vi "FTW-Test-Socket-Stress-InboxConnector.vi"() -> (0 "Test Result":errorcluster)   [LabVIEW 2014]
uses:
  src/core/socket/support/FTW-Socket-Core-TransportScheme.ctl
  src/core/error/FTW-ERR-ExceptionType.ctl
  src/core/error/FTW-ERR-Assert-DeveloperError.vi
  src/core/error/FTW-ERR-ThrowError.vi
  src/core/error/FTW-ERR-CallChain.vi
  src/core/string/FTW-STR-ReplaceWhitespace.vi
panel:
  in  "Mode":enum32{"Automated Testing", "Manual Control"}(tab)
  out "Progress":dbl(slide) scale=0.0..1.0
  in  "Test to Perform":T1(radio)=enum."Parallel: 10x100x10k"
  in  "stop":bool
  out "Results":T3(array[cluster]) {"?" format="%_3p bytes/sec (one-way receive)"; "?" format="%_3f replies/sec"; "?" format="Benchmark Time: %_3psec"}
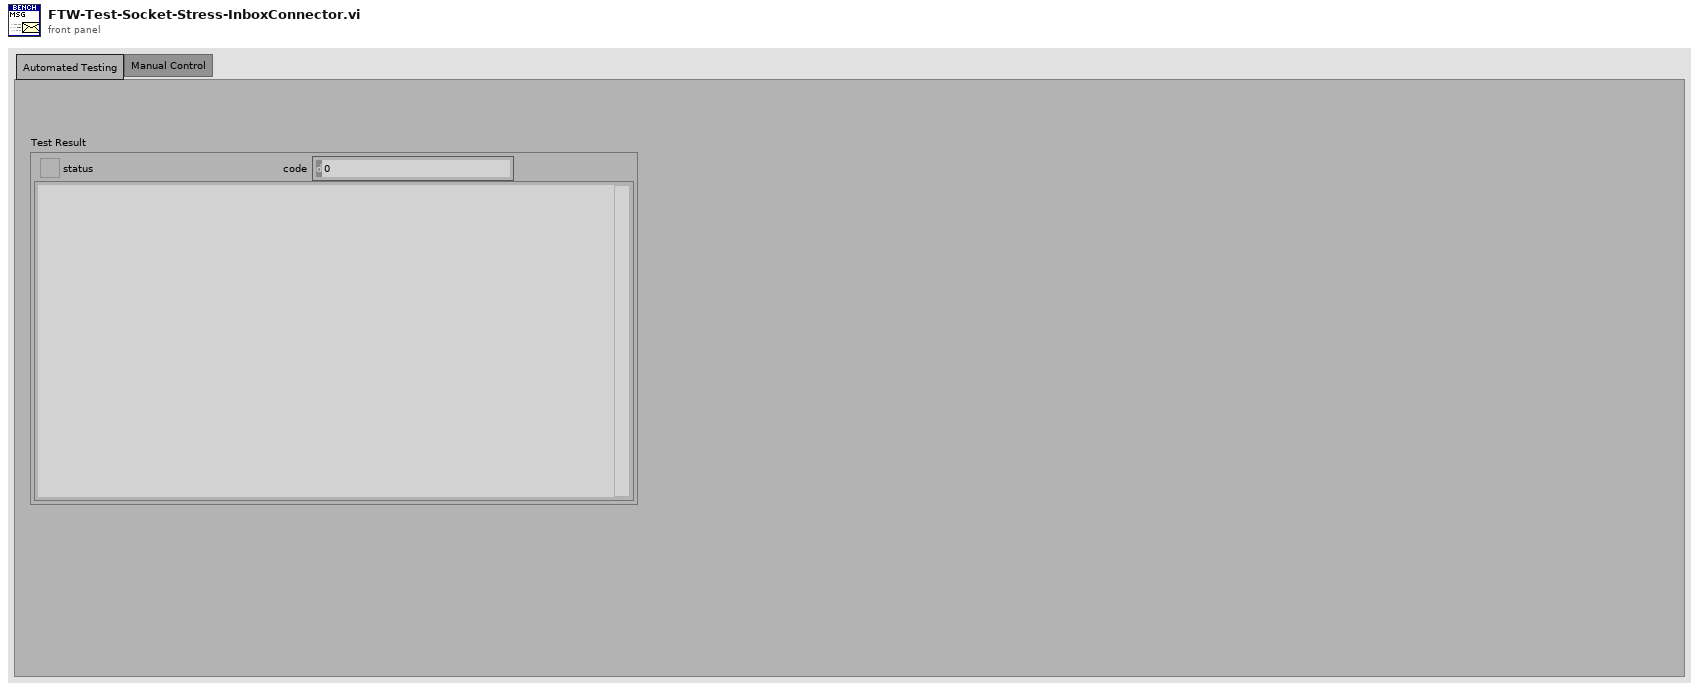
[diagram p1: front panel]
types:
  T1 = enum32{"Serial: 1x1x0", "Serial: 1x1000x0", "Serial: 1x1000x10k", "Serial: 10x100x10k", "Parallel: 10x100x10k", "Parallel: 10x10x1M", "Parallel: 100x1x10k", "Parallel: 100x100x0", "Parallel: 1000x10x1k", "Parallel: 1000x100x10k", "Parallel: 10x100x1M", "Parallel: 1000x1x1M", "Parallel: 10x10000x0"}
  T2 = typedef "FTW-Socket-Core-TransportScheme.ctl" = enum16{"TCP (tcp://)", "Inter-Process (ipc://)", "In-Process (inproc://)", "WebSocket (ws://)"}
  T3 = cluster{"Server Address":T2, "error":errorcluster, "Client Results":cluster{"Instance":string, "All replies were as expected?":bool}[], dbl, dbl, dbl, "Pass?":bool}[]
  T4 = enum32{"Serial: 1x1x0", "Serial: 1x1000x0", "Serial: 1x1000x10k", "Serial: 10x100x10k", "Parallel: 10x100x10k", "Parallel: 10x10x1M", "Parallel: 100x1x10k", "Parallel: 100x100x0", "Parallel: 1000x10x1k", "Parallel: 1000x100x10k", "Parallel: 10x100x1M", "Parallel: 1000x1x1M", "Parallel: 10x10000x0"}[]
  T5 = cluster{"Inbox Address":T2, "error out":errorcluster, cluster{string, bool}[], "Elapsed Time":dbl, dbl, dbl, bool}[]
  T6 = typedef "FTW-ERR-ExceptionType.ctl" = enum16{"OK", "Info", "Warning", "Error"}
  T7 = cluster{i32, i32, i32, i32, "Replies from Server":i32, "bytes from Server":i32, bool, bool}
  T8 = cluster{"Message Transport Scheme":T2, "error out":errorcluster, cluster{string, bool}[], "Elapsed Time":dbl, dbl, dbl, bool}
  T9 = cluster{"Message Transport Scheme":T2, "error out":errorcluster, cluster{string, bool}[], "Elapsed Time":dbl, dbl, dbl, bool}[]
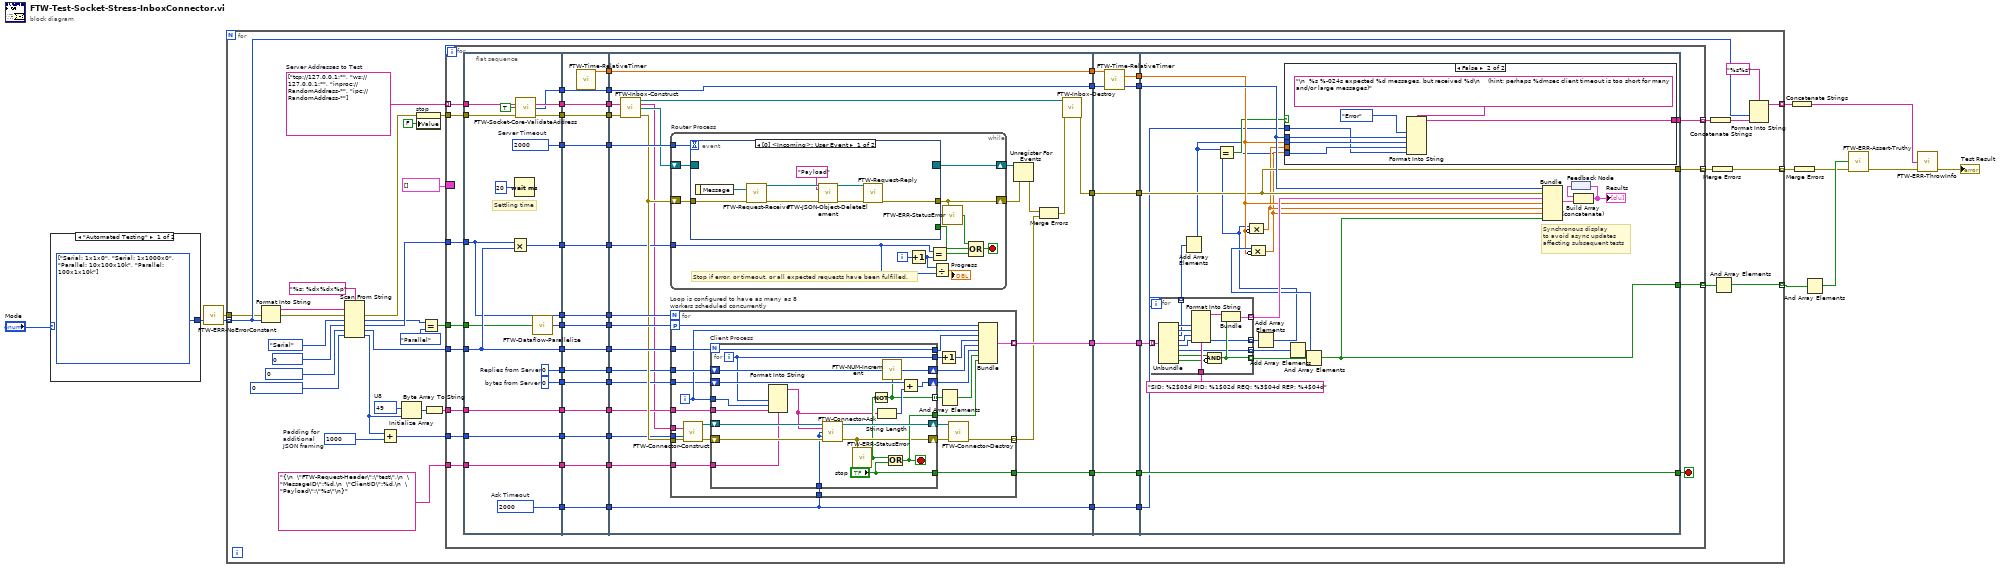
[diagram p0: block diagram]
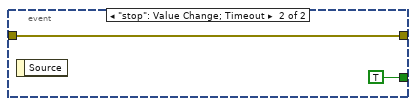
[diagram p2: hidden frame]
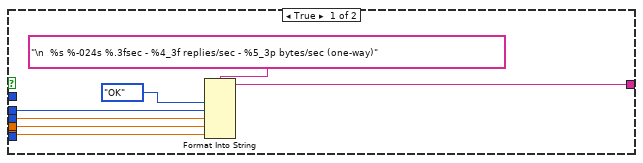
[diagram p3: hidden frame]
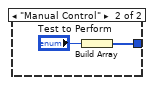
[diagram p4: hidden frame]
diagram:
  n1 = case shown="\"Automated Testing\"" "Mode" {
    tunnel: [w12 w13] -> w10
    frame "Automated Testing" {
      w12 = T4 [enum."Serial: 1x1x0", enum."Serial: 1x1000x0", enum."Parallel: 10x100x10k", enum."Parallel: 100x1x10k"] items=["Serial: 1x1x0", "Serial: 1x1000x0", "Serial: 1x1000x10k", "Serial: 10x100x10k", "Parallel: 10x100x10k", "Parallel: 10x10x1M", "Parallel: 100x1x10k", "Parallel: 100x100x0", "Parallel: 1000x10x1k", "Parallel: 1000x100x10k", "Parallel: 10x100x1M", "Parallel: 1000x1x1M", "Parallel: 10x10000x0"]
    }
    frame "Manual Control" {
      n2 = Build Array("Test to Perform") -> (w13:T4)
    }
  }
  n3 = call "FTW-ERR-NoErrorConstant.vi"() -> ("no error"=w1:errorcluster)
  n4 = for {
    tunnel: w10 -> [w24] mode=indexing
    tunnel: [w40] -> w9 mode=indexing
    tunnel: [w39] -> w8 mode=indexing
    tunnel: [w36] -> w6 mode=indexing
    tunnel: w1 -> [w16]
    w20 = 1000  # Padding for additional JSON framing
    w23 = string[] ["tcp://127.0.0.1:*", "ws://127.0.0.1:*", "inproc://RandomAddress-*", "ipc://RandomAddress-*"]  # Server Addresses to Test
    w46 = u8 49  # U8
    n5 = Format Into String(error in=w16, w24) -> (resulting string=w34:string, error out=w33:errorcluster)  [unwired: 2 in]
    n6 = Scan From String(format string="%s: %dx%dx%p", input string=w34, error in=w33, default 1=enum32{"Parallel", "Serial"}."Serial", default 2=0, default 3=0, default 4=0) -> (error out=w30:errorcluster, output 1=w19:enum32{"Parallel", "Serial"}, output 2=w26:i32, output 3=w25:i32, output 4=w22:i32)  [unwired: 1 in, 2 out]
    n7 = Add(x=w22, y=w20) -> (x+y=w21:i32)
    n8 = Initialize Array(w46, w22) -> (w45:u8[])
    n9 = property on="stop" class="Bool (strict)"(error in=w30, "Value"=FALSE ("stop")) -> (error out=w47:errorcluster)  [unwired: 1 in, 1 out]
    n10 = Equal?(x=w19, y=enum32{"Parallel", "Serial"}."Parallel" ("x")) -> (x = y?=w17:bool)
    n11 = Byte Array To String(unsigned byte array=w45) -> (string=w44:string)
    n12 = for {
      tunnel: w23 -> [w94] mode=indexing
      tunnel: w26 -> [w91]
      tunnel: w25 -> [w87]
      tunnel: w47 -> [w86]
      tunnel: w44 -> [w76]
      border: T5 [] -> [_]
      tunnel: [w63] -> w42 mode=indexing
      tunnel: [w62] -> w41 mode=indexing
      tunnel: [w61] -> w38 mode=indexing
      tunnel: w21 -> [w53]
      tunnel: w17 -> [w52]
      tunnel: "{\n  \"FTW-Request-Header\":\"test\",\n  \"MessageID\":%d,\n  \"ClientID\":%d,\n  \"Payload\":\"%s\"\n}" ("format string") -> [w49]
      stop <- w66 stop-if-true
      n13 = flat-sequence {
        tunnel: [w111] -> w101
        tunnel: [w109] -> w95
        tunnel: [w113] -> w92
        tunnel: [w119] -> w88
        tunnel: w86 -> [w112]
        tunnel: w87 -> [w119]
        tunnel: w91 -> [w113]
        tunnel: w94 -> [w110]
        tunnel: [w115] -> w84
        tunnel: [w104] -> w81
        tunnel: [w118] -> w79
        tunnel: [w117] -> w77
        tunnel: w76 -> [w117]
        tunnel: [w116] -> w74
        tunnel: [w114] -> w68
        tunnel: [w108] -> w59
        tunnel: [w106] -> w56
        tunnel: [w105] -> w54
        tunnel: w53 -> [w105]
        tunnel: w52 -> [w103]
        tunnel: [w102] -> w50
        tunnel: w49 -> [w102]
        tunnel: [w135] -> w100
        tunnel: [w134] -> w99
        tunnel: w101 -> [w135]
        tunnel: [w133] -> w96
        tunnel: w95 -> [w133]
        tunnel: [w132] -> w93
        tunnel: w92 -> [w132]
        tunnel: [w131] -> w89
        tunnel: w88 -> [w131]
        tunnel: [w130] -> w85
        tunnel: w84 -> [w130]
        tunnel: [w123] -> w83
        tunnel: [w129] -> w82
        tunnel: w81 -> [w129]
        tunnel: [w128] -> w80
        tunnel: w79 -> [w128]
        tunnel: [w127] -> w78
        tunnel: w77 -> [w127]
        tunnel: [w126] -> w75
        tunnel: w74 -> [w126]
        tunnel: w68 -> [w125]
        tunnel: [w125] -> w67
        tunnel: [w124] -> w60
        tunnel: w59 -> [w124]
        tunnel: w56 -> [w123]
        tunnel: [w122] -> w55
        tunnel: w54 -> [w122]
        tunnel: [w121] -> w51
        tunnel: w50 -> [w121]
        tunnel: [w148] -> w98
        tunnel: [w162] -> w97
        tunnel: [w161] -> w90
        tunnel: w80 -> [w146]
        tunnel: w82 -> [w155]
        tunnel: w100 -> [w154]
        tunnel: w99 -> [w162]
        tunnel: w96 -> [w153]
        tunnel: w93 -> [w157]
        tunnel: w89 -> [w158]
        tunnel: w85 -> [w156]
        tunnel: w83 -> [w138]
        tunnel: w78 -> [w147]
        tunnel: w75 -> [w144]
        tunnel: [w140] -> w69
        tunnel: w67 -> [w142]
        tunnel: [w141] -> w64
        tunnel: w60 -> [w140]
        tunnel: [w138] -> w57
        tunnel: w55 -> [w137]
        tunnel: w51 -> [w136]
        tunnel: w98 -> [w238]
        tunnel: w97 -> [w237]
        tunnel: w90 -> [w235]
        tunnel: [w238] -> w73
        tunnel: [w236] -> w72
        tunnel: [w235] -> w71
        tunnel: [w234] -> w70
        tunnel: w69 -> [w234]
        tunnel: [w233] -> w65
        tunnel: w64 -> [w233]
        tunnel: [w232] -> w58
        tunnel: w57 -> [w232]
        tunnel: w73 -> [w246]
        tunnel: w72 -> [w248]
        tunnel: w71 -> [w261]
        tunnel: w70 -> [w250]
        tunnel: [w251] -> w66
        tunnel: w65 -> [w251]
        tunnel: [w249] -> w63
        tunnel: [w247] -> w62
        tunnel: [w246] -> w61
        tunnel: w58 -> [w239]
        frame #0 {
          w106 = 2000  # Ask Timeout
          w114 = 0  # bytes from Server
          w115 = 2000  # Server Timeout
          w116 = 0  # Replies from Server
          # "Settling time"
          n14 = Multiply(x=w113, y=w119) -> (x*y=w118:i32)
          n15 = Wait (ms)(milliseconds to wait=u32 20) -> ()  [unwired: 1 out]
          n16 = call "FTW-Socket-Core-ValidateAddress.vi"("Address"=w110, "Allow wildcard replacement?"=TRUE, "error in"=w112) -> ("Sanitized Address"=w109:string, "Message Transport Scheme"=w108:T2, "error out"=w111:errorcluster)  [unwired: 10 in]
          n17 = call "FTW-Dataflow-Parallelize.vi"("Parallelize?"=w103) -> ("Parallel Instances"=w104:i32)
        }
        frame #1 {
          n18 = call "FTW-Time-RelativeTimer.vi"() -> ("Current Time"=w134:dbl)  [unwired: 13 in, 2 out]
        }
        frame #2 {
          n19 = call "FTW-Inbox-Construct.vi"("Primary Inbox Address"=w153, "error in"=w154) -> ("FTW Router"=w152:refnum<data-value>, "Resolved Primary Inbox Address"=w139:string, "Incoming Request"=w145:refnum<event-registration>, "error out"=w151:errorcluster)  [unwired: 10 in]
          n20 = for "Loop is configured to have as many as 8 workers scheduled concurrently" {
            N: w157 -> [_]
            tunnel: w151 -> [w167]
            tunnel: w158 -> [w188]
            tunnel: w138 -> [w187]
            workers-P: w155 -> [w184]
            tunnel: [w186] -> w161 mode=indexing
            tunnel: w139 -> [w168]
            tunnel: [w180] -> w143 mode=indexing
            tunnel: w147 -> [w178]
            tunnel: w144 -> [w177]
            tunnel: w142 -> [w172]
            tunnel: [w170] -> w141
            tunnel: w137 -> [w164]
            tunnel: w136 -> [w163]
            i -> [w175]
            n21 = call "FTW-Connector-Construct.vi"("Remote Inbox Address"=w168, "Receive Message Size Limit"=w164, "error in"=w167) -> ("FTW Actor Connector"=w165:refnum<data-value>, "error out"=w166:errorcluster)  [unwired: 11 in]
            n22 = for "Client Process" {
              N: w188 -> [w196]
              shift-right: [w207] -> w182
              shift-left: w165 -> [w208]
              tunnel: w187 -> [w203]
              tunnel: [w206] -> w185
              tunnel: [w195] -> w179 mode=indexing
              shift-right: [w204] -> w181
              shift-left: w166 -> [w205]
              tunnel: w175 -> [w192]
              tunnel: w178 -> [w191]
              shift-right: [w202] -> w176
              shift-left: w177 -> [w201]
              tunnel: [w193] -> w174
              shift-right: [w199] -> w171
              shift-left: w172 -> [w198]
              tunnel: ["stop"] -> w170
              tunnel: [w196] -> w169
              tunnel: w163 -> [w190]
              i -> [w193]
              stop <- w206 stop-if-true
              n23 = Format Into String(format string=w190, w193, w192, w191) -> (resulting string=w189:string)  [unwired: 2 in, 1 out]
              n24 = call "FTW-Connector-Ask.vi"("FTW Actor Connector"=w208, "Request"=w189, "Receive Timeout"=w203, "Send Timeout"=w203, "error in"=w205) -> ("FTW Actor Connector out"=w207:refnum<data-value>, "error out"=w204:errorcluster)  [unwired: 7 in, 2 out]
              n25 = call "FTW-ERR-StatusError.vi"("error to check"=w204) -> ("Error?"=w194:bool)
              n26 = Not(x=w194) -> (.not. x?=w195:bool)
              n27 = String Length(string=w189) -> (length=w200:i32)
              n28 = call "FTW-NUM-Increment.vi"("Initial Value"=w201, "Increment?"=w195) -> ("Final Value"=w202:i32)
              n29 = Compound Arithmetic op=OR(w194, "stop") -> (w206:bool)
              n30 = Add(x=w198, y=w200) -> (x+y=w199:i32)
            }
            n31 = Increment(x=w174) -> (x+1=w173:i32)
            n32 = And Array Elements(Boolean array=w179) -> (logical AND=w183:bool)
            n33 = call "FTW-Connector-Destroy.vi"("FTW Connector"=w182, "error in"=w181) -> ("error out"=w180:errorcluster)  [unwired: 13 in]
            n34 = Bundle(w184, w175, w169, w173, "Replies from Server"=w176, "bytes from Server"=w171, w183, w185) -> (w186:T7)  [unwired: 1 in]
          }
          n35 = while "Router Process" {
            shift-right: [w220] -> w159
            shift-left: w145 -> [w221]
            shift-right: [w218] -> w160
            shift-left: w151 -> [w219]
            tunnel: w146 -> [w211]
            tunnel: w156 -> [w213]
            i -> [w212]
            stop <- w214 stop-if-true
            # "Stop if error, or timeout, or all expected requests have been fulfilled."
            n36 = event shown="[0] <Incoming>: User Event" {
              selector: w221 -> [_ _]
              dyn-events: [_ _] -> w220
              timeout: w213 -> [_ _]
              tunnel: [_ TRUE] -> w216
              tunnel: w219 -> [w227 w230]
              tunnel: [w229 w230] -> w218
              event User Event {
                n37 = event-data() -> ("Message"=w228:refnum<queue>)  [unwired: 1 in]
                n38 = call "FTW-Request-Receive.vi"("MessagePipe"=w228, "error in"=w227) -> ("Request"=w226:refnum<data-value>, "error out"=w224:errorcluster)  [unwired: 11 in, 1 out]
                n39 = call "FTW-JSON-Object-DeleteElement.vi"("JSON Object"=w226, "Key"="Payload", "error in"=w224) -> ("JSON Object out"=w225:refnum<data-value>, "error out"=w223:errorcluster)  [unwired: 10 in, 1 out]
                n40 = call "FTW-Request-Reply.vi"("Request"=w225, "error in"=w223) -> ("error out"=w229:errorcluster)  [unwired: 13 in]
              }
              event "stop": Value Change; Timeout {
                n41 = event-data() -> ()  [unwired: 1 in, 1 out]
              }
            }
            n42 = Increment(x=w212) -> (x+1=w210:i32)
            n43 = Equal?(x=w211, y=w210) -> (x = y?=w215:bool)
            n44 = Divide(x=w210, y=w211) -> (x/y=→"Progress":dbl)
            n45 = call "FTW-ERR-StatusError.vi"("error to check"=w218) -> ("Error?"=w217:bool)
            n46 = Compound Arithmetic op=OR(w217, w216, w215) -> (w214:bool)
          }
          n47 = Unregister For Events(event registration refnum=w159, error in=w160) -> (error out=w150:errorcluster)
          n48 = Merge Errors(w150, w143) -> (w149:errorcluster)
          n49 = call "FTW-Inbox-Destroy.vi"("FTW Router"=w152, "error in"=w149) -> ("error out"=w148:errorcluster)  [unwired: 13 in]
        }
        frame #3 {
          n50 = call "FTW-Time-RelativeTimer.vi"("Previous Time"=w237) -> ("Elapsed Time"=w236:dbl)  [unwired: 12 in, 2 out]
        }
        frame #4 {
          # "Synchronous display\nto avoid async updates\naffecting subsequent tests"
          n51 = for {
            tunnel: w261 -> [w288] mode=indexing
            tunnel: "SID: %2$03d PID: %1$02d REQ: %3$04d REP: %4$04d" -> [w287]
            tunnel: [w283] -> w258 mode=indexing
            tunnel: [w282] -> w260 mode=indexing
            tunnel: [w279] -> w256 mode=indexing
            tunnel: [w278] -> w252 mode=indexing
            tunnel: [w276] -> w243 mode=indexing
            n52 = Unbundle(w288) -> (w286:i32, w285:i32, w276:i32, w277:i32, "Replies from Server"=w278:i32, "bytes from Server"=w279:i32, w280:bool, w281:bool)
            n53 = Format Into String(format string=w287, w286, w285, w277, w278) -> (resulting string=w284:string)  [unwired: 2 in, 1 out]
            n54 = Compound Arithmetic op=AND(w280, invert w281) -> (w282:bool)
            n55 = Bundle(w284, w282) -> (w283:cluster{string, bool})  [unwired: 1 in]
          }
          n56 = Add Array Elements(numeric array=w243) -> (sum=w241:i32)
          n57 = Add Array Elements(numeric array=w252) -> (sum=w240:i32)
          n58 = Equal?(x=w241, y=w240) -> (x = y?=w242:bool)
          n59 = Compound Arithmetic op=MULTIPLY(w240, invert w248) -> (w245:dbl)
          n60 = Add Array Elements(numeric array=w256) -> (sum=w253:i32)
          n61 = Compound Arithmetic op=MULTIPLY(w253, invert w248) -> (w244:dbl)
          n62 = case shown="False" w242 {
            tunnel: w250 -> [w268 w275]
            tunnel: [w266 w273] -> w249
            tunnel: w248 -> [w265 _]
            tunnel: w245 -> [w264 _]
            tunnel: w244 -> [w263 _]
            tunnel: w241 -> [_ w272]
            tunnel: w240 -> [_ w271]
            tunnel: w239 -> [_ w270]
            frame True {
              n63 = Format Into String(format string="\n  %s %-024s %.3fsec - %4_3f replies/sec - %5_3p bytes/sec (one-way)", FTW-ERR-ExceptionType."OK" ("Exception"), w268, w265, w264, w263) -> (resulting string=w266:string)  [unwired: 2 in, 1 out]
            }
            frame False {
              n64 = Format Into String(format string="\n  %s %-024s expected %d messages, but received %d\n    (hint: perhaps %dmsec client timeout is too short for many and/or large messages)", FTW-ERR-ExceptionType."Error" ("Exception"), w275, w272, w271, w270) -> (resulting string=w273:string)  [unwired: 2 in, 1 out]
            }
          }
          n65 = And Array Elements(Boolean array=w260) -> (logical AND=w247:bool)
          n66 = Bundle("Message Transport Scheme"=w250, "error out"=w246, w258, "Elapsed Time"=w248, w245, w244, w247) -> (w255:T8)  [unwired: 1 in]
          n67 = feedback #1() -> (w259:T5)
          n68 = Build Array (concatenate)(w259, w255) -> (w254:T9)
          "Results" <- w254
          n69 = feedback-in #1(w254) -> ()
        }
      }
    }
    n70 = Concatenate Strings(w42) -> (w37:string)
    n71 = Merge Errors(w38) -> (w39:errorcluster)
    n72 = And Array Elements(Boolean array=w41) -> (logical AND=w40:bool)
    n73 = Format Into String(format string="%s%s", w24, w37) -> (resulting string=w36:string)  [unwired: 2 in, 1 out]
  }
  n74 = Concatenate Strings(w6) -> (w5:string)
  n75 = Merge Errors(w8) -> (w3:errorcluster)
  n76 = And Array Elements(Boolean array=w9) -> (logical AND=w4:bool)
  n77 = call "FTW-ERR-Assert-Truthy.vi"("Expected Truthy"=w4, "error in"=w3) -> ("error out"=w2:errorcluster)  [unwired: 13 in]
  n78 = call "FTW-ERR-ThrowInfo.vi"("Informational Message"=w5, "error in"=w2) -> ("error out"=→"Test Result":errorcluster)  [unwired: 13 in]
